vi "Vision Processing Data.vi"() -> ()   [LabVIEW 2015]
panel:
  out "Distance (ft)":dbl
  out "Bottom of Target":dbl
  out "Top of Target":dbl
  out "Right Side of Target":dbl
  out "Left Side of Target":dbl
  out "Angle X":dbl
  out "Center Y":dbl
  out "Center X":dbl
  out "Sorted Particle Scores":T1(array[cluster]) {"Moment Factor" format="%#_3g"; "Aspect Ratio" format="%#_3g"; "Area to CH" format="%#_3g"; "X" format="%#_3g"; "Y" format="%#_3g"}
  out "Detected Targets":T2(array[cluster]) {"Normalized Rect"."Numeric 5" format="%#_2g"; "Normalized Rect"."Numeric 3" format="%#_2g"; "Normalized Rect"."Numeric 2" format="%#_2g"; "Normalized Rect"."Numeric" format="%#_2g"}
  # "The values are of only one target. I can pull values of more targets if needed, but for right now I think one target is sufficient."
  # "Density Profile"
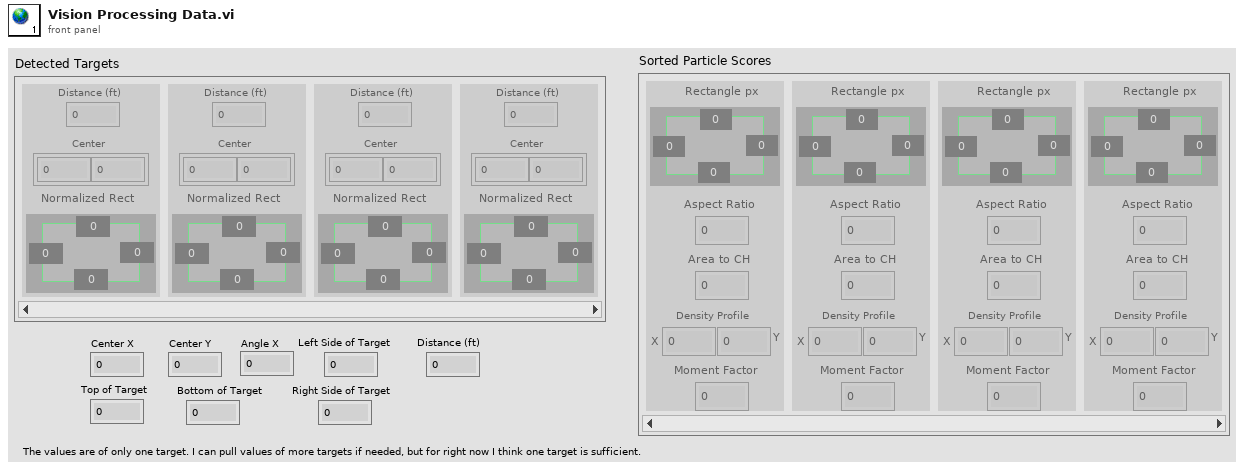
[diagram p1: front panel]
types:
  T1 = cluster{"Rectangle px":cluster{"Numeric":dbl, "Numeric 2":dbl, "Numeric 3":dbl, "Numeric 5":dbl}, "Aspect Ratio":dbl, "Area to CH":dbl, "X":dbl, "Y":dbl, "Moment Factor":dbl}[]
  T2 = cluster{"Distance (ft)":dbl, "Center":cluster{dbl, dbl}, "Normalized Rect":cluster{"Numeric":dbl, "Numeric 2":dbl, "Numeric 3":dbl, "Numeric 5":dbl}}[]
diagram:
